vi "Write Field.vi"(7 "field":string, 8 "error in (no error)":errorcluster, 10 "value":variant, 11 "Base Interface in":refnum<class "Base Interface.lvclass">) -> (0 "error out":errorcluster, 3 "Base Interface out":refnum<class "Base Interface.lvclass">)   [LabVIEW 2020, in "PV Access.lvlib" / "PV Data.lvlib" / "Base Interface.lvclass"]
uses:
  Base Interface.lvclass
  PV Data.lvlib
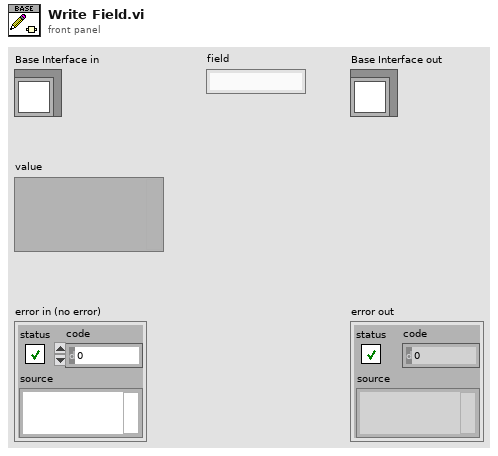
[diagram p1: front panel]
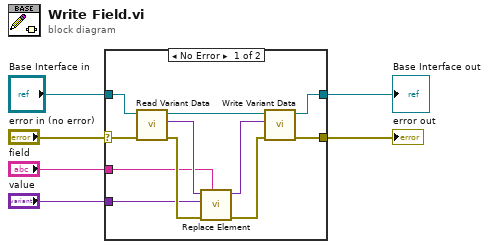
[diagram p0: block diagram]
diagram:
  n1 = case shown="No Error" "error in (no error)" {
    selector: "error in (no error)" -> [w16 w19]
    tunnel: [w15 w19] -> w3
    tunnel: [w13 w18] -> w5
    tunnel: "Base Interface in" -> [w17 w18]
    tunnel: "value" -> [w7 _]
    tunnel: "field" -> [w8 _]
    frame No Error {
      n2 = call-dynamic "Read Variant Data.vi"("error in"=w16, "Base Interface in"=w17) -> ("error out"=w12:errorcluster, "data"=w10:variant, "Base Interface out"=w14:refnum<class "Base Interface.lvclass">)  [unwired: 7 in]
      n3 = call "Replace Element.vi"("element name"=w8, "error in"=w12, "value"=w7, "cluster in"=w10) -> ("error out"=w11:errorcluster, "cluster out"=w9:variant)  [unwired: 6 in]
      n4 = call-dynamic "Write Variant Data.vi"("error in (no error)"=w11, "data"=w9, "Base Interface in"=w14) -> ("error out"=w15:errorcluster, "Base Interface out"=w13:refnum<class "Base Interface.lvclass">)  [unwired: 7 in]
    }
    frame Error {
    }
  }
  "error out" <- w3
  "Base Interface out" <- w5
